vi "E Write cells.vi"(0 "Excel._Worksheet":refnum<k7>, 5 "Cell/表格位置":string, 7 "Array data/二维数组":string[][](array[string]), 11 "error in (no error)":errorcluster) -> (4 "Excel._Worksheet":refnum<k7>, 6 "Excel.Range":refnum<k7>, 15 "error out":errorcluster)   [LabVIEW 2011]
doc: "将数据写进指定的多个单元格里，其中“Cell/表格位置”的格式为“A1：B2”。"
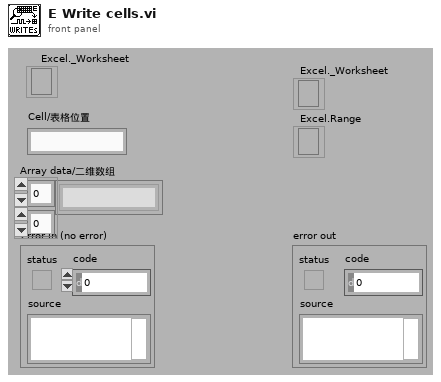
[diagram p1: front panel]
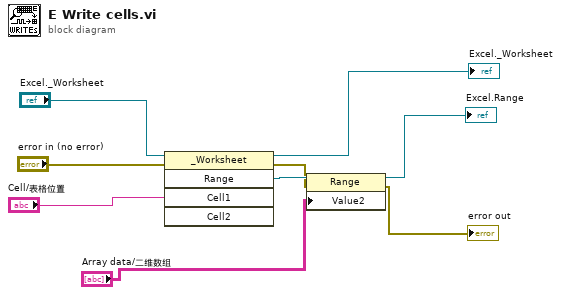
[diagram p0: block diagram]
diagram:
  n1 = invoke class="_Worksheet" method="Range"(reference="Excel._Worksheet", error in="error in (no error)", "Cell1"="Cell/表格位置") -> (reference out=→"Excel._Worksheet":refnum<k7>, error out=w5:errorcluster, "Range"=w6:refnum<k7>)  [unwired: 2 in, 2 out]
  n2 = property class="Range"(reference=w6, error in=w5, "Value2"="Array data/二维数组") -> (reference out=→"Excel.Range":refnum<k7>, error out=→"error out":errorcluster)
